vi "Get Callback Events.vi"(8 "error in (no error)":errorcluster, 11 "SourceGrid in":refnum<class "SourceGrid.lvclass">) -> (0 "error out":errorcluster, 2 "Callback Events":cluster{}, 3 "SourceGrid out":refnum<class "SourceGrid.lvclass">)   [LabVIEW 2024]
uses:
  SourceGrid.lvclass/SourceGrid.ctl
  SourceGrid.lvclass
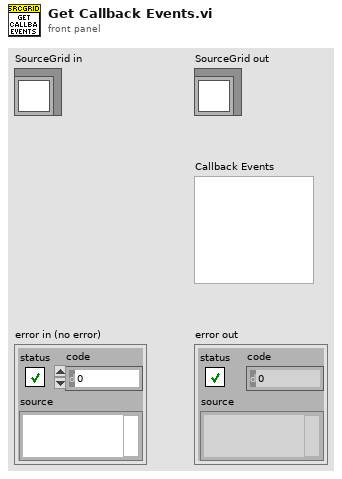
[diagram p1: front panel]
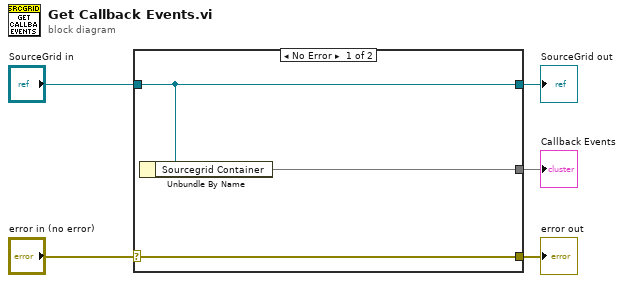
[diagram p0: block diagram]
diagram:
  n1 = case shown="No Error" "error in (no error)" {
    selector: "error in (no error)" -> [w8 w9]
    tunnel: [w8 w9] -> w4
    tunnel: [w7 w10] -> w2
    tunnel: "SourceGrid in" -> [w7 w10]
    tunnel: [w6 _] -> w1
    frame No Error {
      n2 = Unbundle By Name(w7) -> ("Sourcegrid Container"=w6)
    }
    frame Error {
    }
  }
  "error out" <- w4
  "SourceGrid out" <- w2
  "Callback Events" <- w1
